vi "Read RepoType.vi"(8 "error in (no error)":errorcluster, 11 "Package in":refnum<class "Package.lvclass">) -> (0 "error out":errorcluster, 2 "RepoType":T1, 3 "Package out":refnum<class "Package.lvclass">)   [LabVIEW 2016, in "Packages.lvlib" / "Package.lvclass"]
uses:
  Package.lvclass
  Repo_class/RepoType--enum.ctl
  Package.lvclass/Package.ctl
  Repo_class/Repo.lvclass
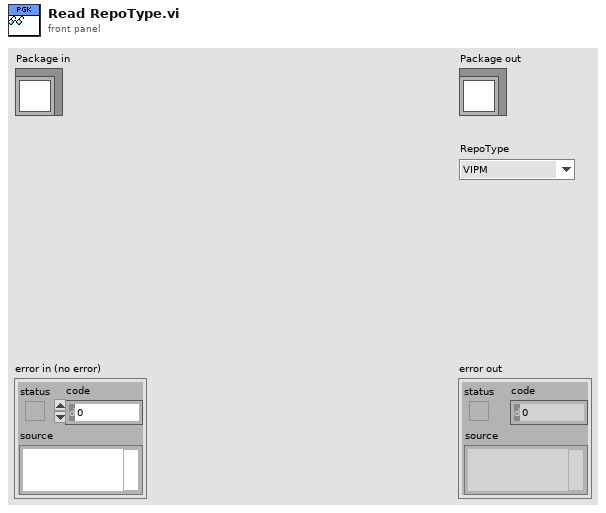
[diagram p1: front panel]
types:
  T1 = typedef "Packages.lvlib/Repo.lvclass/RepoType--enum.ctl" = enum16{"VIPM", "NIPM", "GPM"}
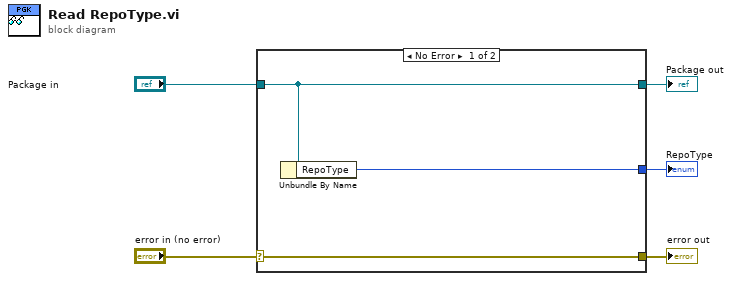
[diagram p0: block diagram]
diagram:
  n1 = case shown="No Error" "error in (no error)" {
    selector: "error in (no error)" -> [w8 w9]
    tunnel: [w8 w9] -> w4
    tunnel: [w7 w10] -> w2
    tunnel: "Package in" -> [w7 w10]
    tunnel: [w6 _] -> w1
    frame No Error {
      n2 = Unbundle By Name(w7) -> ("RepoType"=w6:T1)
    }
    frame Error {
    }
  }
  "error out" <- w4
  "Package out" <- w2
  "RepoType" <- w1
